vi "Dialog_Setup Filter String.vi"(7 "Action":T1, 8 "error in":errorcluster, 11 "Filter String Ref":refnum<vi>) -> (0 "error out":errorcluster, 3 "Filter String Ref Out":refnum<vi>)   [LabVIEW 2023]
uses:
  controls/action enum.ctl
panel:
  in  "Filter":string
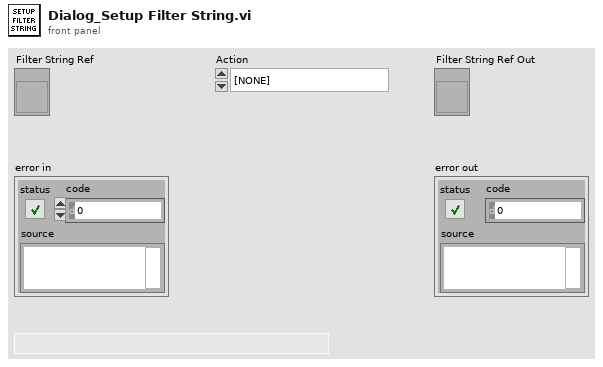
[diagram p1: front panel]
types:
  T1 = typedef "action enum.ctl" = enum16{"[NONE]", "Wire Bundle", "Wire Unbundle", "Terminal Unbundle", "Terminal Bundle", "Bundler Move Up", "Bundler Move Down", "Bundler Insert", "Bundler Remove", "Bundler Remove Unwired", "Bundler Rearrange", "In Place Insert", "In Place Remove", "In Place Remove Unwired", "In Place Rearrange", "Wire Properties", "Wire Method", "Terminal Properties", "Terminal Method", "Property Move Up", "Property Move Down", "Properties Insert", "Properties Remove", "Properties Remove Unwired", "Properties Rearrange", "Method Change", "Class for Constant", "Class For Control", "Class For Node", "Class Name to Clipboard"}
  T2 = enum16{"[NONE]", "Wire Bundle", "Wire Unbundle", "Terminal Unbundle", "Terminal Bundle", "Bundler Insert", "Bundler Remove", "Bundler Remove Unwired", "Bundler Rearrange", "In Place Insert", "In Place Remove", "In Place Remove Unwired", "In Place Rearrange", "Wire Properties", "Wire Method", "Terminal Properties", "Terminal Method", "Properties Insert", "Properties Remove", "Properties Remove Unwired", "Properties Rearrange", "Method Change", "Class for Constant", "Class For Control", "Class For Node", "Class Name to Clipboard"}
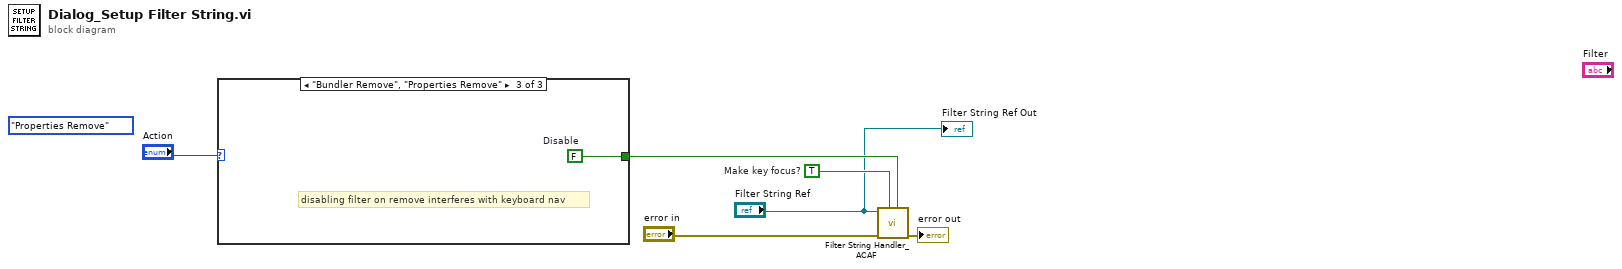
[diagram p0: block diagram]
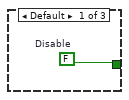
[diagram p2: hidden frame]
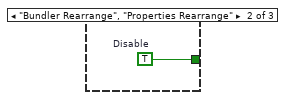
[diagram p3: hidden frame]
diagram:
  (unwired) T2."Properties Remove" ("Action")
  w6 = TRUE  # Make key focus?
  n1 = case shown="\"Bundler Remove\", \"Properties Remove\"" "Action" {
    tunnel: [w7 w8 w9] -> w3
    frame Default {
      w7 = FALSE  # Disable
    }
    frame "Bundler Rearrange", "Properties Rearrange" {
      w8 = TRUE  # Disable
    }
    frame "Bundler Remove", "Properties Remove" {
      w9 = FALSE  # Disable
      # "disabling filter on remove interferes with keyboard nav"
    }
  }
  n2 = call "Filter String Handler_ACAF.vi"("Disable"=w3, "Make key focus?"=w6, "error in (no error)"="error in", "String Ref"="Filter String Ref") -> ("error out"=→"error out":errorcluster)  [unwired: 7 in]
  "Filter String Ref Out" <- "Filter String Ref"
